vi "TP Editor-Save AS.vi"(0 "Program path":path, 3 "error in (no error)":errorcluster, 6 "File Name":string) -> (7 ".not. x?":bool, 8 "Cancel":bool, 9 "File Name 2":string, 10 "error out":errorcluster)   [LabVIEW 2018]
panel:
  in  "Cancel":bool
  in  "OK":bool
  in  "Program list":i32(listbox)
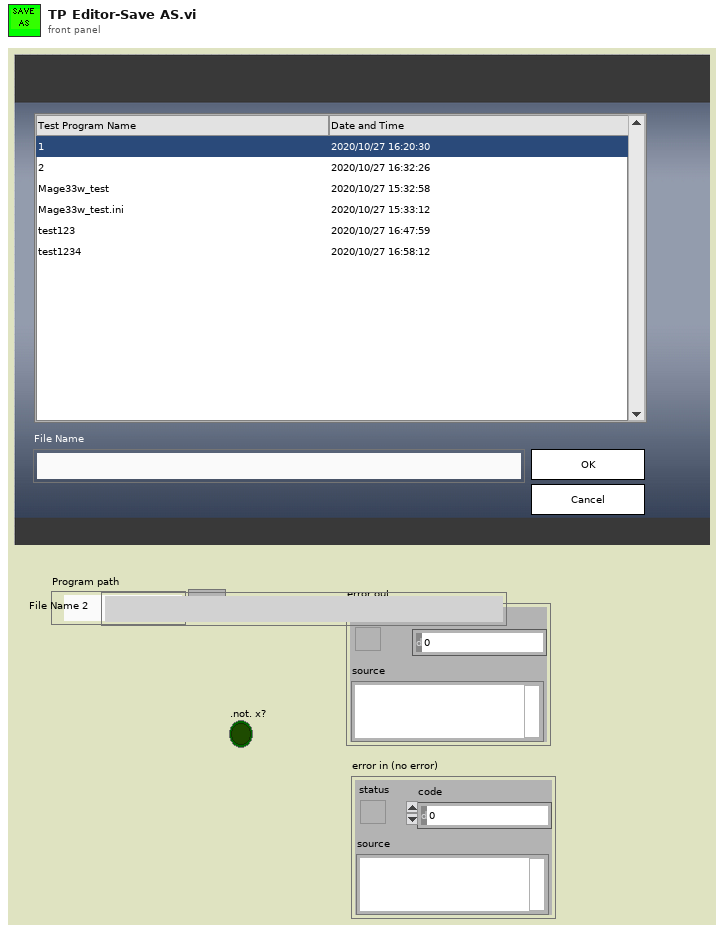
[diagram p1: front panel]
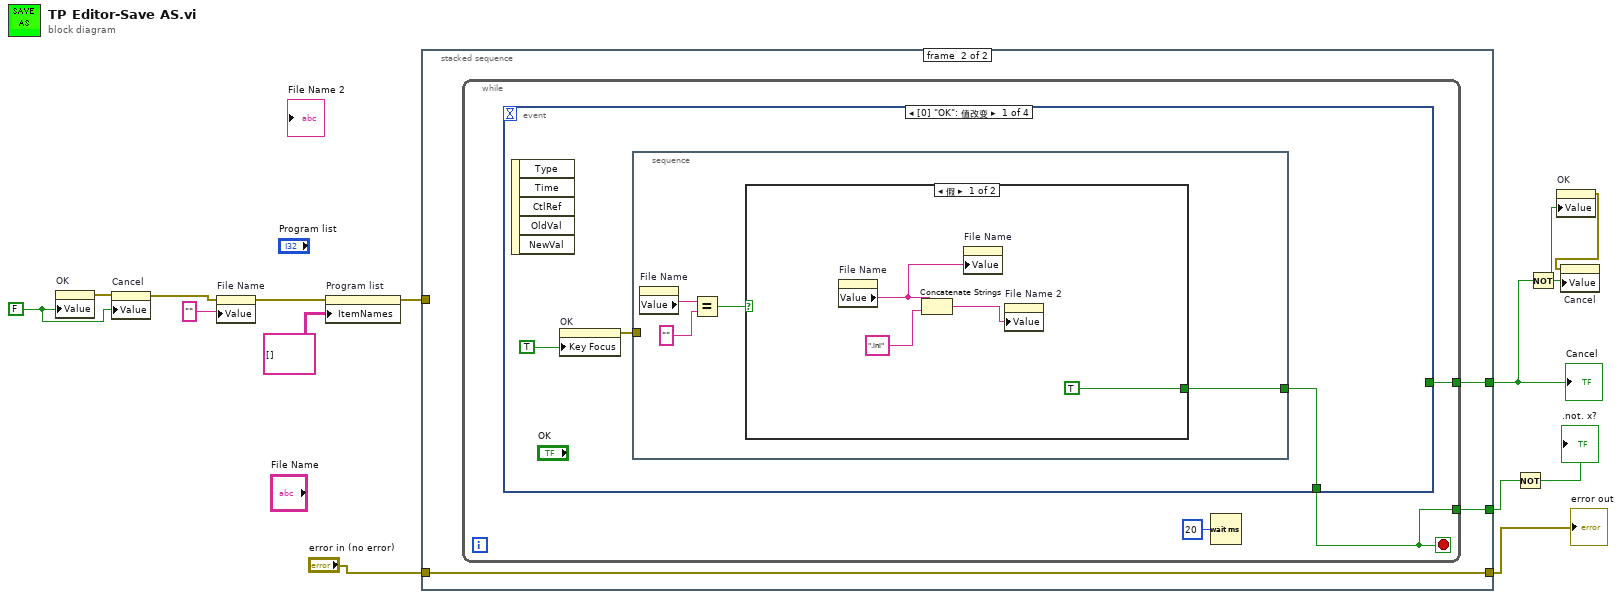
[diagram p0: block diagram]
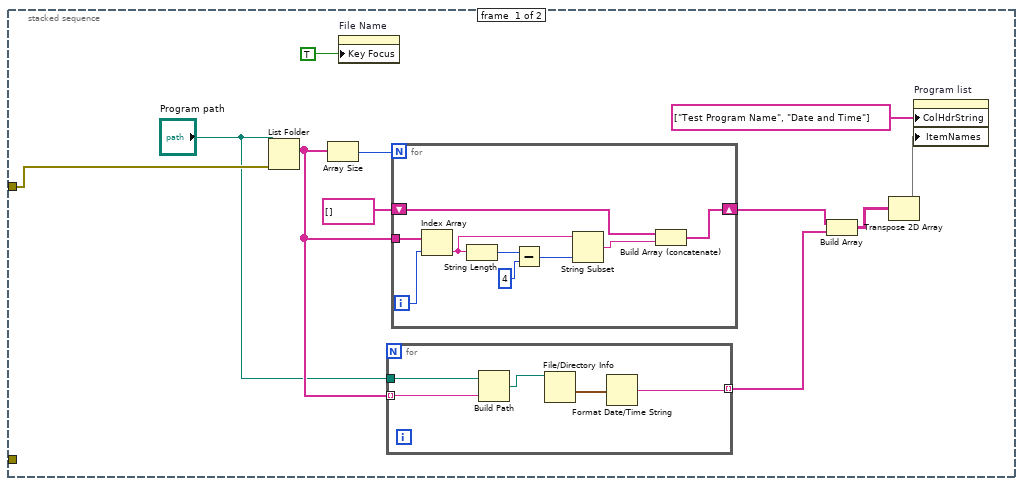
[diagram p2: hidden frame]
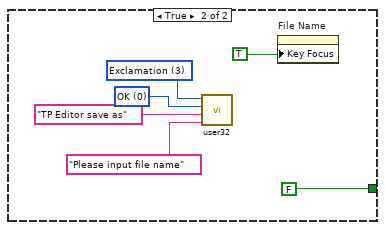
[diagram p3: hidden frame]
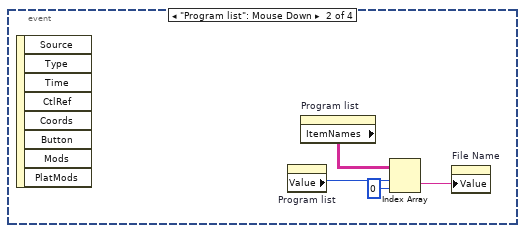
[diagram p4: hidden frame]
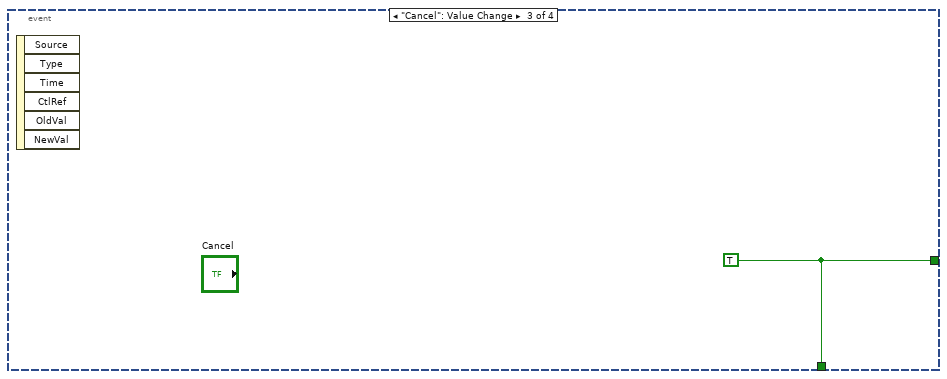
[diagram p5: hidden frame]
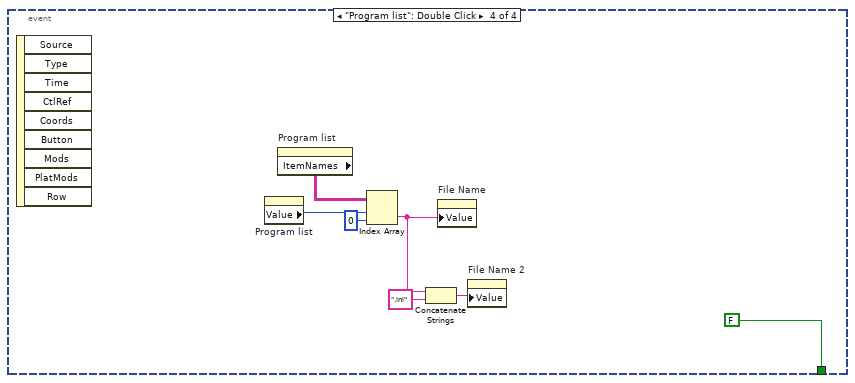
[diagram p6: hidden frame]
diagram:
  w1 = FALSE
  n1 = property on="OK" class="Bool (严格)"("Value"=w1) -> (error out=w3:errorcluster)  [unwired: 2 in, 1 out]
  n2 = property on="Cancel" class="Bool (严格)"(error in=w3, "Value"=w1) -> (error out=w2:errorcluster)  [unwired: 1 in, 1 out]
  n3 = property on="File Name" class="Str"(error in=w2, "Value"="") -> (error out=w11:errorcluster)  [unwired: 1 in, 1 out]
  n4 = property on="Program list" class="MCListbox (严格)"(error in=w11, "ItemNames"=string[][] []) -> (error out=w13:errorcluster)  [unwired: 1 in, 1 out]
  n5 = stacked-sequence {
    tunnel: [_ w42] -> w9
    tunnel: w13 -> [w20 _]
    tunnel: [_ w41] -> w10
    tunnel: "error in (no error)" -> [_ w41]
    tunnel: [_ w40] -> w6
    frame #0 {
      n6 = List Folder(path="Program path", error in=w20) -> (filenames=w19:string[])  [unwired: 5 out]
      n7 = Array Size(array=w19) -> (size(s)=w24:i32)
      n8 = property on="File Name" class="Str"("Key Focus"=TRUE) -> ()  [unwired: 2 in, 2 out]
      n9 = for {
        tunnel: w19 -> [w29] mode=indexing
        tunnel: "Program path" -> [w30]
        tunnel: [w26] -> w17 mode=indexing
        n10 = Build Path(base path=w30, name or relative path=w29) -> (appended path=w28:path)
        n11 = File/Directory Info(path=w28) -> (last mod=w27:timestamp)  [unwired: 1 in, 6 out]
        n12 = Format Date/Time String(seconds (now)=w27) -> (date/time string=w26:string)  [unwired: 2 out]
      }
      n13 = for {
        N: w24 -> [_]
        tunnel: w19 -> [w39]
        shift-right: [w32] -> w15
        shift-left: string[] [] -> [w31]
        i -> [w38]
        n14 = Index Array(array=w39, index=w38) -> (element=w35:string)
        n15 = String Length(string=w35) -> (length=w37:i32)
        n16 = Subtract(x=w37, y=4) -> (x-y=w34:i32)
        n17 = String Subset(string=w35, length (rest)=w34) -> (substring=w33:string)  [unwired: 1 out]
        n18 = Build Array (concatenate)(w31, w33) -> (w32:string[])
      }
      n19 = Build Array(w15, w17) -> (w16:string[][])
      n20 = Transpose 2D Array(2D array=w16) -> (transposed array=w22:string[][])
      n21 = property on="Program list" class="MCListbox (严格)"("ColHdrString"=string[] ["Test Program Name", "Date and Time"] ("Column Header Strings[]"), "ItemNames"=w22) -> ()  [unwired: 2 in, 2 out]
    }
    frame #1 {
      n22 = while {
        tunnel: [w44] -> w42
        tunnel: [w43] -> w40
        stop <- w44 stop-if-true
        n23 = event shown="[0] \"OK\": 值改变" {
          selector: _ -> [_ _ _ _]
          dyn-events: _ -> [_ _ _ _]
          timeout: _ -> [_ _ _ _]
          tunnel: [w48 _ w67 FALSE] -> w44
          tunnel: [_ _ w67 _] -> w43
          event "OK": Value Change {
            n24 = event-data() -> ()  [unwired: 6 out]
            n25 = property on="OK" class="Bool (严格)"("Key Focus"=TRUE) -> (error out=w47:errorcluster)  [unwired: 2 in, 1 out]
            n26 = stacked-sequence {
              tunnel: [w49] -> w48
              tunnel: w47 -> [_]
              frame #0 {
                n27 = property on="File Name" class="Str"() -> ("Value"=w52:string)  [unwired: 2 in, 2 out]
                n28 = Equal?(x=w52, y="") -> (x = y?=w50:bool)
                n29 = case shown="假" w50 {
                  tunnel: [TRUE FALSE] -> w49
                  frame False {
                    n30 = property on="File Name" class="Str"() -> ("Value"=w54:string)  [unwired: 2 in, 2 out]
                    n31 = Concatenate Strings(w54, ".ini" ("string")) -> (w53:string)
                    n32 = property on="File Name" class="Str"("Value"=w54) -> ()  [unwired: 2 in, 2 out]
                    n33 = property on="File Name 2" class="Str"("Value"=w53) -> ()  [unwired: 2 in, 2 out]
                  }
                  frame True {
                    w61 = u16 0 items=["OK", "OK+Cancel", "Abort+Retry+Ignore", "Yes+ON+Cancel", "Yes+No", "Retry+Cancel", "Cancel+Retry+Continue"] ("Buttons")
                    w62 = u16 3 items=["None", "Critical", "Question", "Exclamation", "Infomation"] ("Icon")
                    n34 = call "user32.vi"("Icon"=w62, "Buttons"=w61, "Ipcaption"="TP Editor save as", "IP Text"="Please input file name") -> ()  [unwired: 2 out]
                    n35 = property on="File Name" class="Str"("Key Focus"=TRUE) -> ()  [unwired: 2 in, 2 out]
                  }
                }
              }
            }
          }
          event "Program list": Mouse Down {
            n36 = event-data() -> ()  [unwired: 9 out]
            n37 = property on="Program list" class="MCListbox (严格)"() -> ("Value"=w65:i32)  [unwired: 2 in, 2 out]
            n38 = property on="Program list" class="MCListbox (严格)"() -> ("ItemNames"=w66:string[][])  [unwired: 2 in, 2 out]
            n39 = Index Array(array=w66, index (row)=w65, index (col)=0 ("disabled index (col)")) -> (element=w63:string)
            n40 = property on="File Name" class="Str"("Value"=w63) -> ()  [unwired: 2 in, 2 out]
          }
          event "Cancel": Value Change {
            w67 = TRUE
            n41 = event-data() -> ()  [unwired: 7 out]
          }
          event "Program list": Double Click {
            n42 = event-data() -> ()  [unwired: 10 out]
            n43 = property on="Program list" class="MCListbox (严格)"() -> ("Value"=w73:i32)  [unwired: 2 in, 2 out]
            n44 = property on="Program list" class="MCListbox (严格)"() -> ("ItemNames"=w74:string[][])  [unwired: 2 in, 2 out]
            n45 = Index Array(array=w74, index (row)=w73, index (col)=0 ("disabled index (col)")) -> (element=w69:string)
            n46 = Concatenate Strings(w69, ".ini" ("string")) -> (w70:string)
            n47 = property on="File Name" class="Str"("Value"=w69) -> ()  [unwired: 2 in, 2 out]
            n48 = property on="File Name 2" class="Str"("Value"=w70) -> ()  [unwired: 2 in, 2 out]
          }
        }
        n49 = Wait (ms)(milliseconds to wait=u32 20) -> ()  [unwired: 1 out]
      }
    }
  }
  "error out" <- w10
  "Cancel" <- w6
  n50 = Not(x=w9) -> (.not. x?=→".not. x?":bool)
  n51 = Not(x=w6) -> (.not. x?=w5:bool)
  n52 = property on="OK" class="Bool (严格)"("Value"=w5) -> (error out=w4:errorcluster)  [unwired: 2 in, 1 out]
  n53 = property on="Cancel" class="Bool (严格)"(error in=w4, "Value"=w5) -> ()  [unwired: 1 in, 2 out]
